vi "read data (SubVI).vi"() -> (2 "DATA's boolean":bool[](array[boolean]), 3 "read  data":u8 format="%b")   [LabVIEW 2019]
uses:
  <vilib>/rvi/eio/common/nirviEmuTemplateMethod_errors.vi
  <vilib>/eio/EIONode/EIONode.xnode
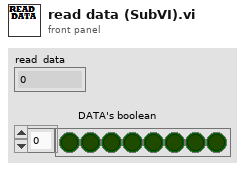
[diagram p1: front panel]
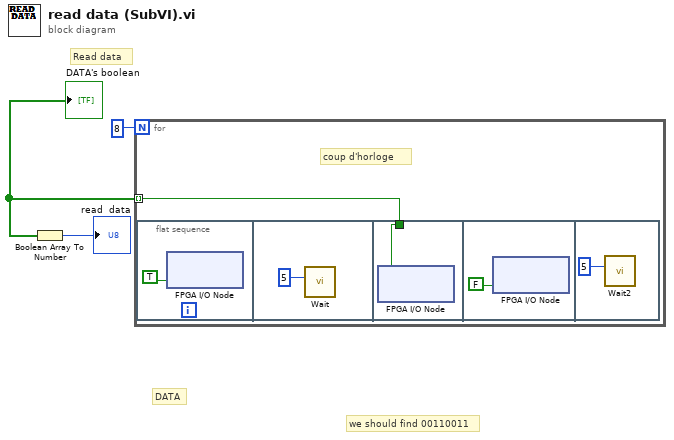
[diagram p0: block diagram]
diagram:
  # "we should find 00110011"
  # "DATA"
  # "Read data"
  n1 = for {
    N: 8 -> [_]
    tunnel: [w4] -> w2 mode=indexing
    # "coup d'horloge"
    n2 = flat-sequence {
      tunnel: [w7] -> w4
      frame #0 {
        n3 = xnode "FPGA I/O Node"("SCL"=TRUE) -> ()  [unwired: 1 in, 1 out]
      }
      frame #1 {
        n4 = call "Wait"("Count(uSec)"=u32 5 ("Count(Ticks)")) -> ()  [unwired: 1 out]
      }
      frame #2 {
        n5 = xnode "FPGA I/O Node"() -> ("SDA"=w7:bool)  [unwired: 1 in, 1 out]
      }
      frame #3 {
        n6 = xnode "FPGA I/O Node"("SCL"=FALSE) -> ()  [unwired: 1 in, 1 out]
      }
      frame #4 {
        n7 = call "Wait2"("Count(uSec)"=u32 5 ("Count(Ticks)")) -> ()  [unwired: 1 out]
      }
    }
  }
  "DATA's boolean" <- w2
  n8 = Boolean Array To Number(Boolean array=w2) -> (number=→"read  data":u8)
